vi "get elapsed time.vi"(8 "error in":errorcluster) -> (0 "error out":errorcluster, 1 "time spent paused (seconds)":dbl format="%.3f", 2 "time spent running (seconds)":dbl format="%.3f", 3 "time elapsed since start (seconds)":dbl format="%.3f")   [LabVIEW 2020, in "main.lvlib" / "stopwatch_timer.lvlib"]
uses:
  stopwatch_timer.lvlib
  library_variable.vi
panel:
  # "Development\ncontrols/indicators useful for development and testing, but which are not outputs of the VI"
  # "Input\nInputs to the VI"
  # "Output\nOutputs of the VI"
  # "Description\n\nBlank VI with error handling case. \n\nSummarize the use of this VI in this space."
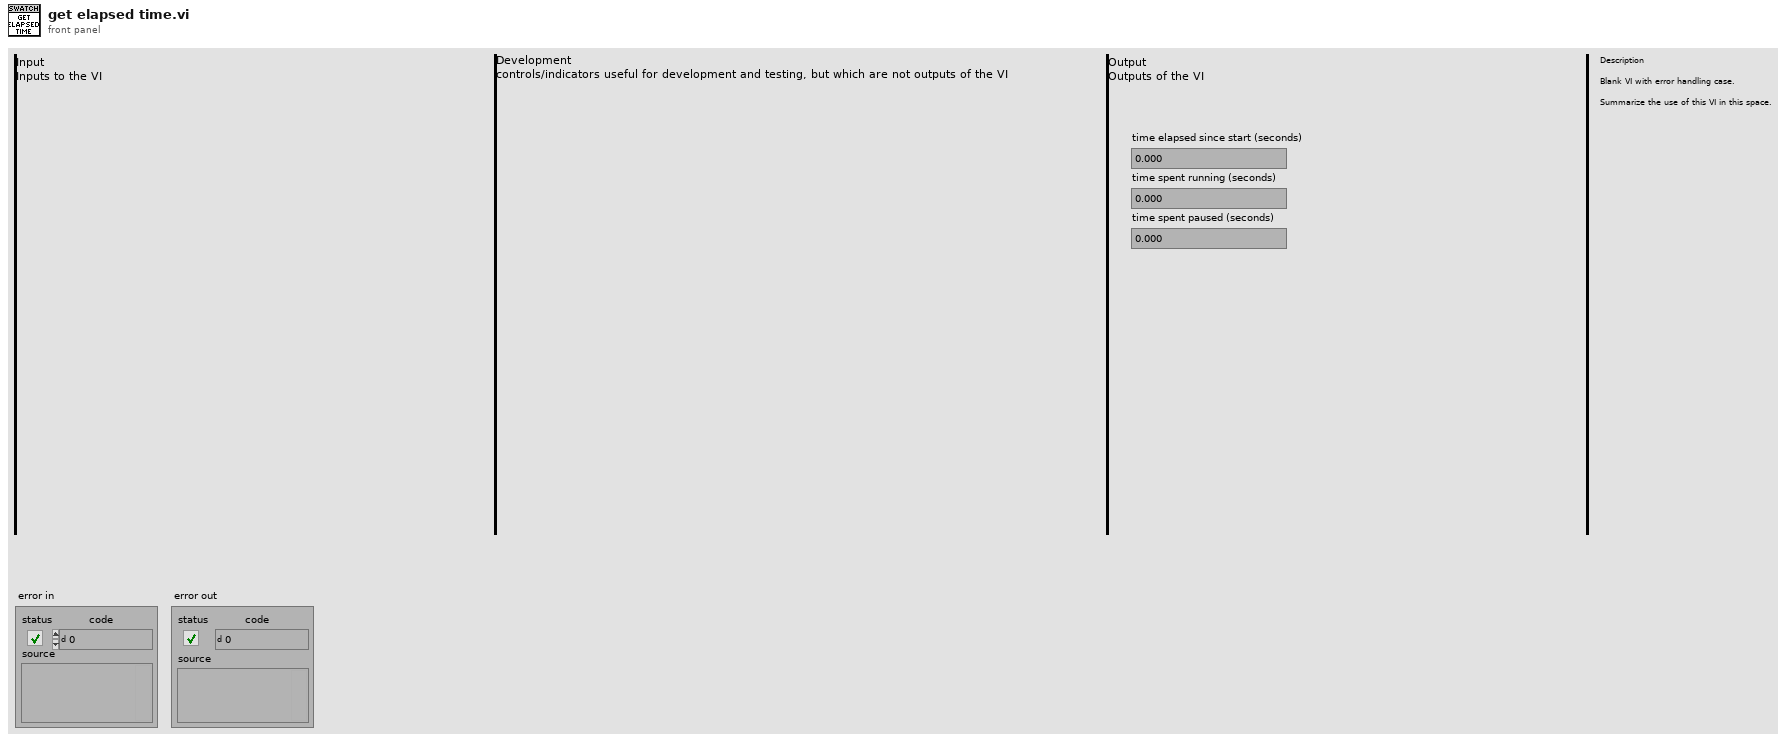
[diagram p1: front panel]
types:
  T1 = typedef "main.lvlib/stopwatch_timer.lvlib/stopwatch data.ctl" = cluster{"state":T2, "started at":timestamp, "last resumed at":timestamp, "last paused at":timestamp, "total time running (seconds)":dbl, "total time paused (seconds)":dbl}
  T2 = typedef "main.lvlib/stopwatch_timer.lvlib/state.ctl" = enum16{"not started", "running", "paused"}
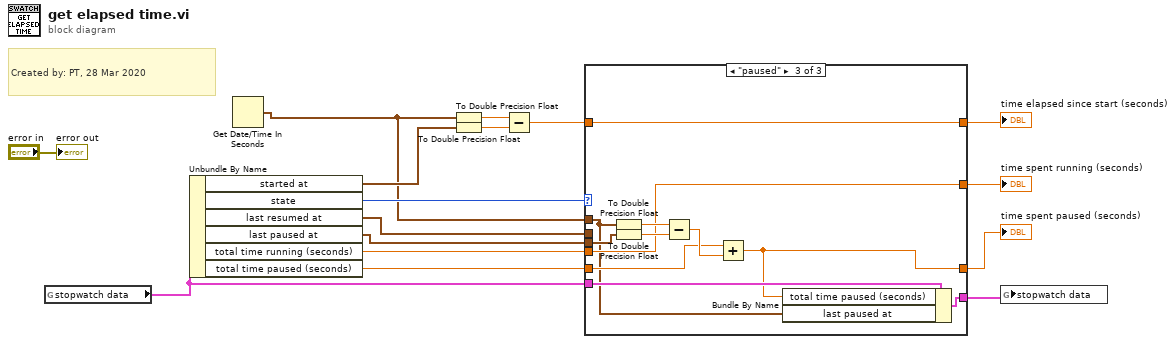
[diagram p0: block diagram]
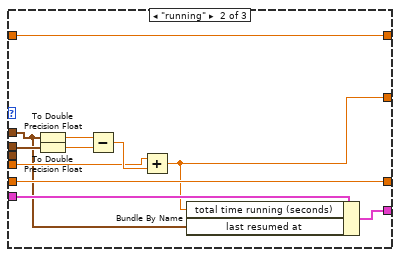
[diagram p3: hidden frame]
diagram:
  # "Created by: PT, 28 Mar 2020"
  n1 = global read "library_variable.vi" "stopwatch data"() -> (w2:T1)
  n2 = Unbundle By Name(w2) -> ("started at"=w14:timestamp, "state"=w15:T2, "last resumed at"=w11:timestamp, "last paused at"=w5:timestamp, "total time running (seconds)"=w10:dbl, "total time paused (seconds)"=w7:dbl)
  n3 = Get Date/Time In Seconds() -> (seconds since 1Jan1904=w9:timestamp)
  n4 = To Double Precision Float(number=w9) -> (double precision float=w13:dbl)
  n5 = To Double Precision Float(number=w14) -> (double precision float=w12:dbl)
  n6 = Subtract(x=w13, y=w12) -> (x-y=w3:dbl)
  n7 = case shown="\"paused\"" w15 {
    tunnel: w11 -> [_ w26 _]
    tunnel: w10 -> [_ w20 w35]
    tunnel: w9 -> [_ w18 w29]
    tunnel: [_ w19 w35] -> w8
    tunnel: w7 -> [_ w24 w31]
    tunnel: [_ w24 w30] -> w6
    tunnel: w5 -> [_ _ w36]
    tunnel: [_ w23 w34] -> w4
    tunnel: w3 -> [_ w23 w34]
    tunnel: w2 -> [w17 w22 w33]
    tunnel: [w17 w21 w32] -> w1
    frame "not started" {
    }
    frame "running" {
      n8 = To Double Precision Float(number=w18) -> (double precision float=w27:dbl)
      n9 = To Double Precision Float(number=w26) -> (double precision float=w28:dbl)
      n10 = Subtract(x=w27, y=w28) -> (x-y=w25:dbl)
      n11 = Add(x=w20, y=w25) -> (x+y=w19:dbl)
      n12 = Bundle By Name(cluster=w22, "total time running (seconds)"=w19, "last resumed at"=w18) -> (w21:T1)
    }
    frame "paused" {
      n13 = To Double Precision Float(number=w29) -> (double precision float=w38:dbl)
      n14 = To Double Precision Float(number=w36) -> (double precision float=w39:dbl)
      n15 = Subtract(x=w38, y=w39) -> (x-y=w37:dbl)
      n16 = Add(x=w31, y=w37) -> (x+y=w30:dbl)
      n17 = Bundle By Name(cluster=w33, "total time paused (seconds)"=w30, "last paused at"=w29) -> (w32:T1)
    }
  }
  "time elapsed since start (seconds)" <- w4
  "time spent running (seconds)" <- w8
  "time spent paused (seconds)" <- w6
  n18 = global write "library_variable.vi" "stopwatch data"(w1) -> ()
  "error out" <- "error in"
